vi "GET Channels.vi"(7 "Channel Direction":string, 8 "error in (no error)":errorcluster, 11 "Item Ref in":T1 format="%.0x") -> (0 "error out":errorcluster, 3 "VS Channel Array":refnum<class "ChannelVS.lvclass">[](array[class]))   [LabVIEW 2020, in "Shared Variables CD 2.0 Configuration.lvlib" / "ChannelVS.lvclass"]
uses:
  ChannelVS.lvclass
  <vilib>/NI VeriStand/Custom Device API/Custom Device Item Ref.ctl
  Public/Documents/National Instruments/NI VeriStand 2020/Custom Devices/Shared Variables CD 2.0/data/Channel.lvlibp/1abvi3w/vi.lib/Utility/Data Type/Type Definitions/Data Type.ctl
  ChannelVS.lvclass/ChannelVS.ctl
  Shared/SV Global.vi
  <vilib>/NI VeriStand/Custom Device API/Get Item Property (String).vi
  <vilib>/NI VeriStand/Custom Device API/Get Item Property (Variant).vi
  <vilib>/NI VeriStand/Custom Device API/Custom Device API.lvlib
  Public/Documents/National Instruments/NI VeriStand 2020/Custom Devices/Shared Variables CD 2.0/data/Channel.lvlibp/Channel.lvclass
  Public/Documents/National Instruments/NI VeriStand 2020/Custom Devices/Shared Variables CD 2.0/data/Channel.lvlibp/1abvi3w/vi.lib/Utility/Data Type/NI_Data Type.lvlib
  C:/Users/Public/Documents/National Instruments/NI VeriStand 2020/Custom Devices/Shared Variables CD 2.0/data/Channel.lvlibp/Channel.lvclass
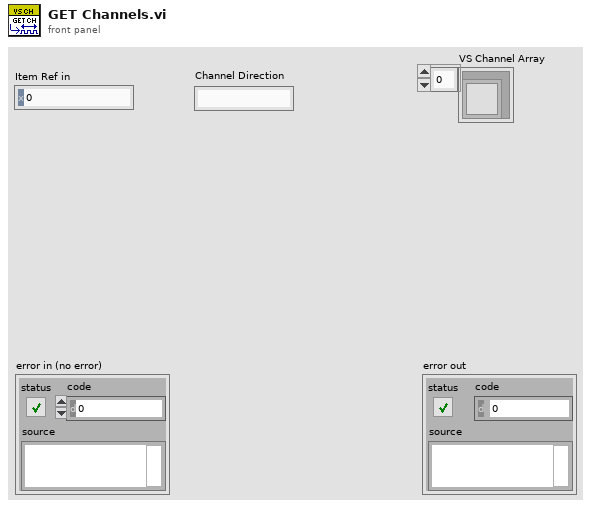
[diagram p1: front panel]
types:
  T1 = typedef "Custom Device API.lvlib/Custom Device Item Ref.ctl" = u64
  T2 = typedef "Channel.lvlibp/NI_Data Type.lvlib/Data Type.ctl" = enum8{"Invalid Type", "Void", "I8", "I16", "I32", "I64", "U8", "U16", "U32", "U64", "Single Float", "Double Float", "Extended Float", "Single Complex", "Double Complex", "Extended Complex", "Enum U8", "Enum U16", "Enum U32", "Enum U64", "Single Float With Unit", "Double Float With Unit", "Extended Float With Unit", "Single Complex with Unit", "Double Complex with Unit", "Extended Complex with Unit", "Boolean", "String", "Path", "Picture", "Tag", "Array", "Cluster", "Variant", "LV Variant", "Waveform", "Timestamp", "Digital Waveform", "Digital Data", "ExpressData", "Refnum", "External Data", "VI", "Poly VI", "LabVIEW Class Instance", "Fixed Point", "Set Collection", "Map Collection"}
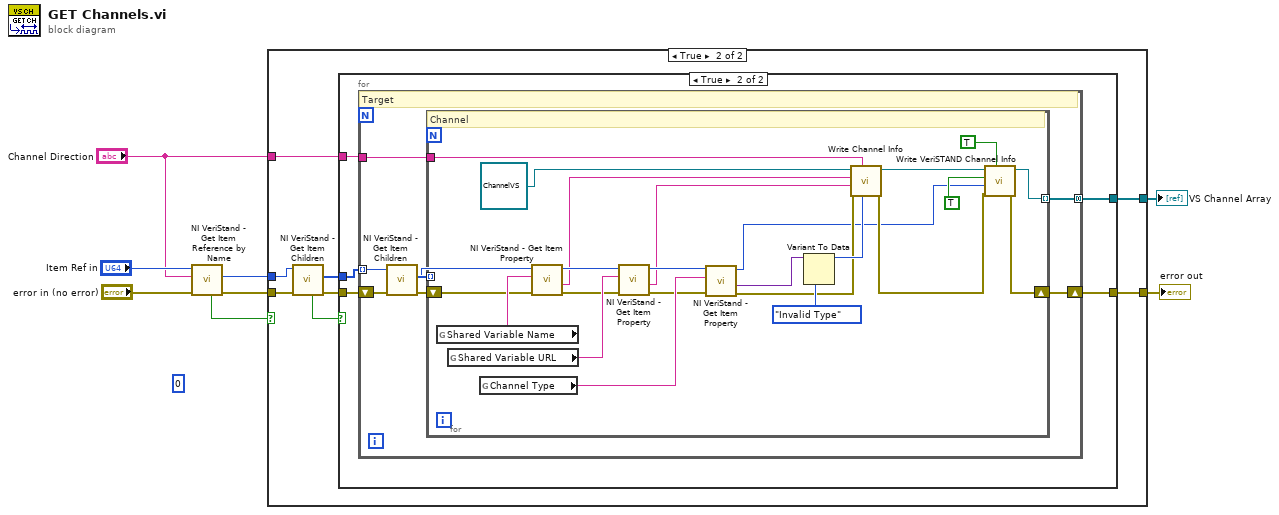
[diagram p0: block diagram]
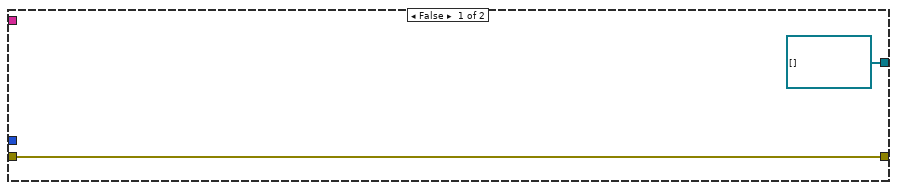
[diagram p2: hidden frame]
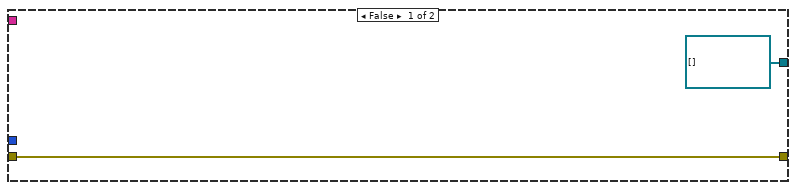
[diagram p3: hidden frame]
diagram:
  (unwired) T1 0 ("Item Ref in")
  n1 = call <vilib>:"NI VeriStand - Get Item Reference by Name.vi"("error in (no error)"="error in (no error)", "Item Name"="Channel Direction", "Parent Ref in"="Item Ref in") -> ("error out"=w5:errorcluster, "Item Ref"=w4:T1, "Found"=w2:bool)  [unwired: 5 in, 1 out]
  n2 = case shown="True" w2 {
    tunnel: [w10 w18] -> w8
    tunnel: [refnum<class "ChannelVS.lvclass">[] [] w15] -> w1
    tunnel: w5 -> [w10 w14]
    tunnel: w4 -> [_ w13]
    tunnel: "Channel Direction" -> [_ w12]
    frame False {
    }
    frame True {
      n3 = call <vilib>:"NI VeriStand - Get Item Children.vi"("error in (no error)"=w14, "Item Ref in"=w13) -> ("error out"=w17:errorcluster, "Child Refs"=w16:T1[], "Found"=w11:bool)  [unwired: 6 in, 1 out]
      n4 = case shown="True" w11 {
        tunnel: [w20 w25] -> w18
        tunnel: w17 -> [w20 w24]
        tunnel: w16 -> [_ w23]
        tunnel: [refnum<class "ChannelVS.lvclass">[] [] w22] -> w15
        tunnel: w12 -> [_ w21]
        frame False {
        }
        frame True {
          n5 = for {
            tunnel: w23 -> [w32] mode=indexing
            shift-right: [w28] -> w25
            shift-left: w24 -> [w30]
            tunnel: [w27] -> w22 mode=concatenating
            tunnel: w21 -> [w26]
            # "Target"
            n6 = call <vilib>:"NI VeriStand - Get Item Children.vi"("error in (no error)"=w30, "Item Ref in"=w32) -> ("error out"=w29:errorcluster, "Child Refs"=w31:T1[])  [unwired: 6 in, 2 out]
            n7 = for {
              tunnel: w31 -> [w37] mode=indexing
              shift-right: [w38] -> w28
              shift-left: w29 -> [w51]
              tunnel: [w40] -> w27 mode=indexing
              tunnel: w26 -> [w45]
              # "Channel"
              n8 = global read "SV Global.vi" "Shared Variable Name"() -> (w56:string)
              n9 = global read "SV Global.vi" "Shared Variable URL"() -> (w54:string)
              n10 = global read "SV Global.vi" "Channel Type"() -> (w53:string)
              n11 = call-poly <vilib>:"NI VeriStand - Get Item Property.vi"("error in (no error)"=w51, "Property Name"=w56, "Item Ref in"=w37) -> ("error out"=w50:errorcluster, "Value"=w47:string, "Item Ref out"=w55:T1)  [unwired: 5 in, 1 out]
              n12 = call-poly <vilib>:"NI VeriStand - Get Item Property.vi"("error in (no error)"=w50, "Property Name"=w54, "Item Ref in"=w55) -> ("error out"=w49:errorcluster, "Value"=w46:string, "Item Ref out"=w52:T1)  [unwired: 5 in, 1 out]
              n13 = call-poly <vilib>:"NI VeriStand - Get Item Property.vi"("error in (no error)"=w49, "Property Name"=w53, "Item Ref in"=w52) -> ("error out"=w41:errorcluster, "Value"=w48:variant, "Item Ref out"=w36:T1)  [unwired: 5 in, 1 out]
              n14 = Variant To Data(type=Data_Type."Invalid Type" ("DataType"), Variant=w48) -> (data=w43:T2)  [unwired: 1 in, 1 out]
              n15 = call "Write Channel Info.vi"("DataType"=w43, "Read or Write"=w45, "error in (no error)"=w41, "URL"=w46, "Name"=w47, "Channel in"=refnum<class "ChannelVS.lvclass"> refnum ("Shared Variables CD 2.0 Configuration.lvlib:ChannelVS.lvclass")) -> ("error out"=w39:errorcluster, "Channel out"=w34:refnum<class "ChannelVS.lvclass">)  [unwired: 4 in]
              n16 = call "Write VeriSTAND Channel Info.vi"("Supported in CD"=TRUE, "error in (no error)"=w39, "VeriSTAND Reference"=w36, "Exist in VeriSTAND"=TRUE, "ChannelVS in"=w34) -> ("error out"=w38:errorcluster, "ChannelVS out"=w40:refnum<class "ChannelVS.lvclass">)  [unwired: 5 in]
            }
          }
        }
      }
    }
  }
  "error out" <- w8
  "VS Channel Array" <- w1
